vi "InsertUndeclaredItem.vi"(8 "error in (no error)":errorcluster, 9 "ILabVIEWItem":refnum<class "ILabVIEWItem.lvclass">, 11 "CReporter in":refnum<class "CReporter.lvclass">) -> (0 "error out":errorcluster, 3 "CReporter out":refnum<class "CReporter.lvclass">)   [LabVIEW 2020, in "DependencyInspection.lvlib" / "CReporter.lvclass"]
uses:
  CReporter.lvclass
  obj/Addons/LabVIEWObjectInterfaces.lvlibp/LabVIEWObjectInterfaces/ILabVIEWItem/ILabVIEWItem.lvclass
  CReporter.lvclass/CReporter.ctl
  CDependencyList/CDependencyList.lvclass
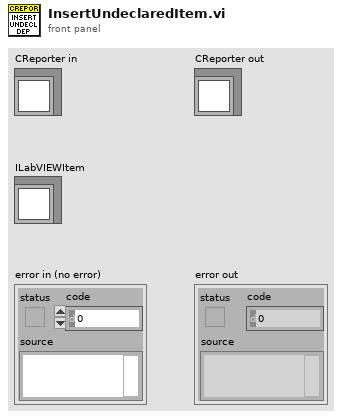
[diagram p1: front panel]
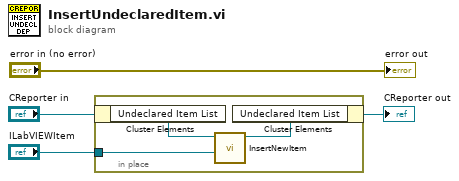
[diagram p0: block diagram]
diagram:
  n1 = in-place {
    in-place-border: "ILabVIEWItem" -> [w6]
    n2 = in-place-cluster #1("CReporter in") -> ("Undeclared Item List"=w7:refnum<class "CDependencyList.lvclass">)
    n3 = call-dynamic "InsertNewItem.vi"("ILabVIEWItem in"=w6, "CDependencyList in"=w7) -> ("CDependencyList out"=w5:refnum<class "CDependencyList.lvclass">)  [unwired: 7 in, 2 out]
    n4 = in-place-cluster #1("Undeclared Item List"=w5) -> (→"CReporter out":refnum<class "CReporter.lvclass">)
  }
  "error out" <- "error in (no error)"
